vi "Read wrapnum.vi"(8 "error in (no error)":errorcluster, 11 "CableWrapCommands in":refnum<class "CableWrapCommands.lvclass">) -> (0 "error out":errorcluster, 2 "wrapnum":T1, 3 "CableWrapCommands out":refnum<class "CableWrapCommands.lvclass">)   [LabVIEW 2014, in "TCSDataDefinitions.lvlib" / "TCSCommand.lvlib" / "CableWrapCommands.lvlib" / "CableWrapCommands.lvclass"]
uses:
  CableWrapCommands.lvclass
  Enumerations/WrapnumTypes.ctl
  CableWrapCommands.lvclass/CableWrapCommands.ctl
  CableWrapCommands.lvlib
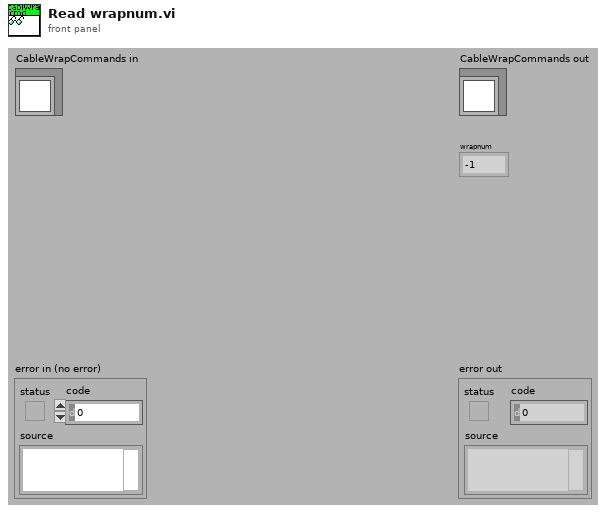
[diagram p1: front panel]
types:
  T1 = typedef "TCSDataDefinitions.lvlib/TCSCommand.lvlib/CableWrapCommands.lvlib/WrapnumTypes.ctl" = enum16{"-1", "0", "1"}
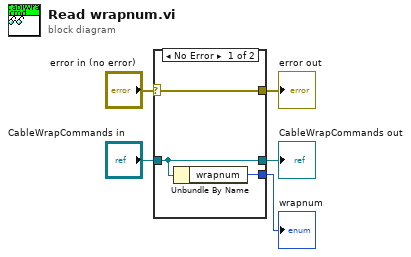
[diagram p0: block diagram]
diagram:
  n1 = case shown="No Error" "error in (no error)" {
    selector: "error in (no error)" -> [w8 w9]
    tunnel: [w8 w9] -> w4
    tunnel: [w7 w10] -> w2
    tunnel: "CableWrapCommands in" -> [w7 w10]
    tunnel: [w6 _] -> w1
    frame No Error {
      n2 = Unbundle By Name(w7) -> ("wrapnum"=w6:T1)
    }
    frame Error {
    }
  }
  "error out" <- w4
  "CableWrapCommands out" <- w2
  "wrapnum" <- w1
